vi "Get Data.vi"(11 "ExpFitter in":refnum<class "ExpFitter.lvclass">) -> (2 "DataExpFit":T1)   [LabVIEW 2019, in "ExpFitter.lvclass"]
uses:
  ExpFitter.lvclass
  TypeDef/DataExpFit.ctl
  ExpFitter.lvclass/ExpFitter.ctl
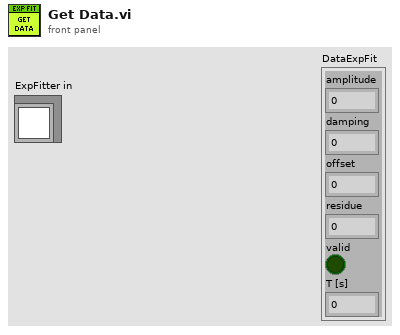
[diagram p1: front panel]
types:
  T1 = typedef "DataExpFit.ctl" = cluster{"amplitude":dbl, "damping":dbl, "offset":dbl, "residue":dbl, "valid":bool, "T [s]":dbl}
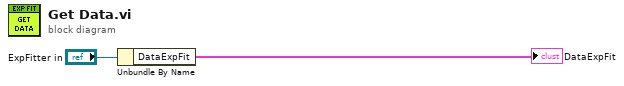
[diagram p0: block diagram]
diagram:
  n1 = Unbundle By Name("ExpFitter in") -> ("DataExpFit"=→"DataExpFit":T1)
